vi "Acknowledge.vi"(7 "ack":refnum<k4>, 10 "parms in":T2={"subchannel"=0, "size (0)"=0, "abort (F)"=FALSE, "timeout"=-1, "ack id (0)"=0, "last elt? (F)"=FALSE, "valid? (T)"=FALSE, "GUID"=""}, 11 "MessengerMCPU in":refnum<class "MessengerMCPU.lvclass">) -> (2 "parms out":T1, 3 "MessengerMCPU out":refnum<class "MessengerMCPU.lvclass">)   [LabVIEW 2019, in "MessengerM.lvlib" / "MessengerMCPU.lvclass"]
uses:
  MessengerMCPU.lvclass
  ParmsOut.ctl
  MessengerM.lvlib
  ParmsIn.ctl
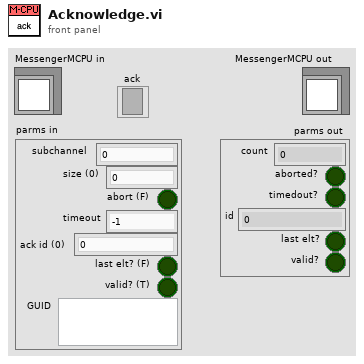
[diagram p1: front panel]
types:
  T1 = typedef "MessengerM.lvlib/ParmsOut.ctl" = cluster{"count":i32, "aborted?":bool, "timedout?":bool, "id":u32, "last elt?":bool, "valid?":bool}
  T2 = typedef "MessengerM.lvlib/ParmsIn.ctl" = cluster{"subchannel":i32, "size (0)":i32, "abort (F)":bool, "timeout":i32, "ack id (0)":u32, "last elt? (F)":bool, "valid? (T)":bool, "GUID":string}
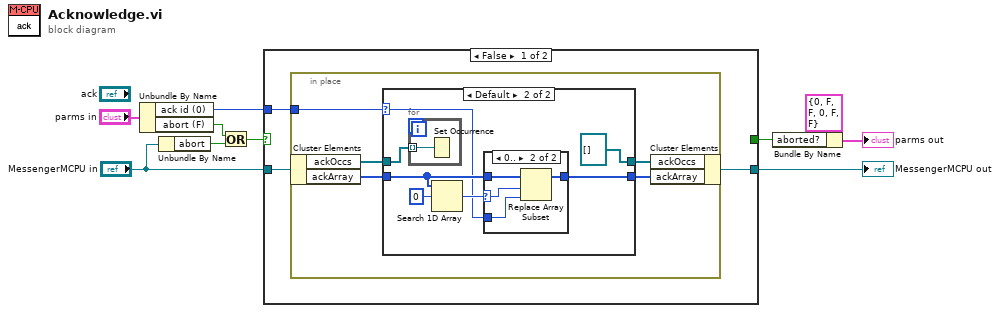
[diagram p0: block diagram]
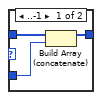
[diagram p3: hidden frame]
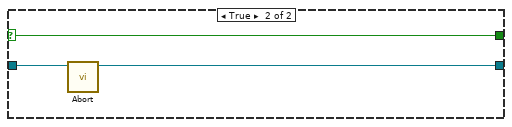
[diagram p4: hidden frame]
diagram:
  n1 = Unbundle By Name("parms in") -> ("ack id (0)"=w4:u32, "abort (F)"=w5:bool)
  n2 = Unbundle By Name("MessengerMCPU in") -> ("abort"=w8:bool)
  n3 = Or(x=w5, y=w8) -> (x .or. y?=w7:bool)
  n4 = case shown="False" w7 {
    selector: w7 -> [_ w38]
    tunnel: [w13 w36] -> w10
    tunnel: "MessengerMCPU in" -> [w12 w37]
    tunnel: [_ w38] -> w2
    tunnel: w4 -> [w11 _]
    frame False {
      n5 = in-place {
        in-place-border: w11 -> [w14]
        n6 = in-place-cluster #1(w12) -> ("ackOccs"=w16:refnum<k4>[], "ackArray"=w18:u32[])
        n7 = case shown="Default" w14 {
          selector: w14 -> [_ w23]
          tunnel: w18 -> [w20 w27]
          tunnel: [w20 w26] -> w17
          tunnel: w16 -> [w19 w22]
          tunnel: [w19 refnum<k4>[] [] ("ackOccs")] -> w15
          frame 0 {
          }
          frame Default {
            n8 = for {
              tunnel: w22 -> [w28] mode=indexing
              n9 = Set Occurrence(w28) -> ()
            }
            n10 = Search 1D Array(1D array=w27, element=u32 0) -> (index of element=w25:i32)  [unwired: 1 in]
            n11 = case shown="0.." w25 {
              selector: w25 -> [_ w33]
              tunnel: [w30 w34] -> w26
              tunnel: w27 -> [w31 w35]
              tunnel: w23 -> [w29 w32]
              frame ..-1 {
                n12 = Build Array (concatenate)(w31, w29) -> (w30:u32[])
              }
              frame 0.. {
                n13 = Replace Array Subset(array=w35, new element=w32, index=w33) -> (w34:u32[])
              }
            }
          }
        }
        n14 = in-place-cluster #1("ackOccs"=w15, "ackArray"=w17) -> (w13:refnum<class "MessengerMCPU.lvclass">)
      }
    }
    frame True {
      n15 = call-dynamic "Abort.vi"("MessengerMCPU in"=w37) -> ("MessengerMCPU out"=w36:refnum<class "MessengerMCPU.lvclass">)  [unwired: 10 in]
    }
  }
  "MessengerMCPU out" <- w10
  n16 = Bundle By Name(cluster=T1 {"count"=0, "aborted?"=FALSE, "timedout?"=FALSE, "id"=0, "last elt?"=FALSE, "valid?"=FALSE} ("parms out"), "aborted?"=w2) -> (→"parms out":T1)
